vi "Poly_SetServo.vi"   [LabVIEW 2012]
doc: "Sets the Servo wired to the specified \"Port\" according to \"Variable in\", to be set as follows:\n1 ms is all the way in one direction\n2 ms is all the way in the other direction\n1.5 ms is in the middle"
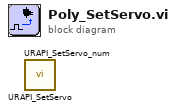
[diagram p0: block diagram]
diagram:
  n1 = call <userlib>:"URAPI_SetServo.vi"() -> ()  [unwired: 4 in, 2 out]
  n2 = call <userlib>:"URAPI_SetServo_num.vi"() -> ()  [unwired: 4 in, 2 out]
